vi "build-flow-controller.vi"(10 "Proc Name":string, 11 "Device":T1={"Schedular"={"sched-mode"=enum."Hourly", "sched-pairs"=[]}, "Sensor"={"Input"="ain", "Comparison"=">=", "Setpoint"=0.0}, "Outputs"=[], "Interval"=0, "Timeout"=0, "Mode"=enum."On"} caption="Device Setup" {"Schedular"."sched-pairs"."start" format="%<%H:%M %d/%m>T"; "Schedular"."sched-pairs"."stop" format="%<%H:%M %d/%m>T"; "Timeout" min=1}) -> (3 "Flow":T7[](array[typedef]))   [LabVIEW 2024]
uses:
  controls/UiStepBuilder.ctl
  controls/type.step-builder.ctl
  controls/controller.ctl
  controls/sched-cluster.ctl
  controls/UiScheduleTimestamp.ctl
  controls/UiDeviceSensorParams.ctl
  controls/UiDeviceSensorEquality.ctl
  controls/device-mode.ctl
  controls/typeFlowBuilderDeviceGenerics.ctl
  controls/sched-encoded-cluster.ctl
panel:
  out "error out":errorcluster
  # "Pulse [sec]"
  # "Period [sec]"
  # "Sensor"
  # "Scheduler"
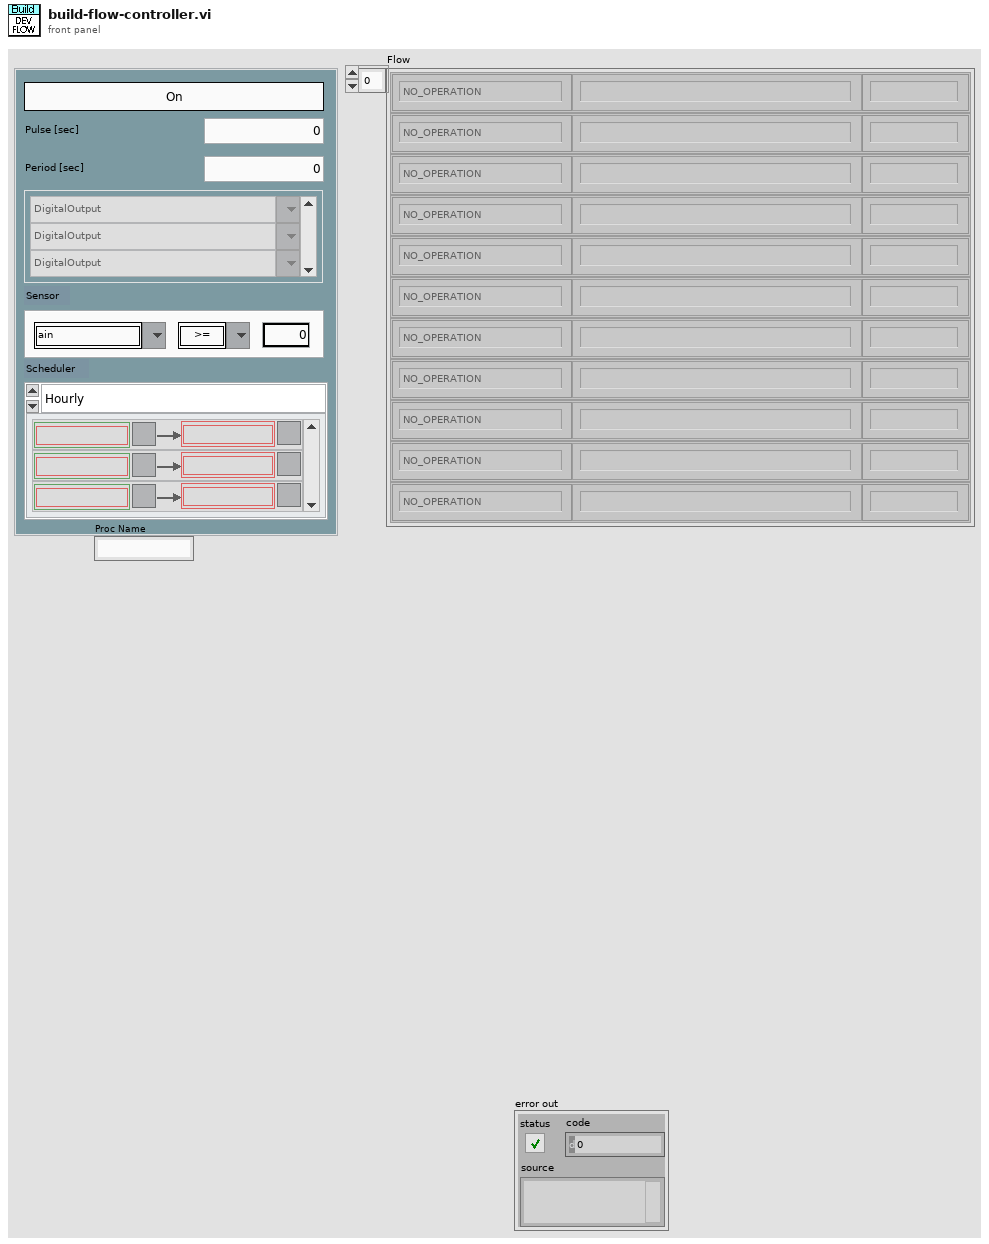
[diagram p1: front panel]
types:
  T1 = typedef "controller.ctl" = cluster{"Schedular":T2, "Sensor":T4, "Outputs":string[], "Interval":u32, "Timeout":u16, "Mode":T6}
  T2 = typedef "sched-cluster.ctl" = cluster{"sched-mode":enum16{"Hourly", "Daily", "Weekly", "Date"}, "sched-pairs":cluster{"start":T3, "stop":T3}[]}
  T3 = typedef "UiScheduleTimestamp.ctl" = timestamp
  T4 = typedef "UiDeviceSensorParams.ctl" = cluster{"Input":string, "Comparison":T5, "Setpoint":dbl}
  T5 = typedef "UiDeviceSensorEquality.ctl" = string
  T6 = typedef "device-mode.ctl" = enum16{"On", "Off", "Sense", "Sched", "Sched AND Sense", "Sched OR Sense"}
  T7 = typedef "UiStepBuilder.ctl" = cluster{"Step Function":T8, "ParamString":string, "Step Label":string}
  T8 = typedef "type.step-builder.ctl" = enum16{"NO_OPERATION", "DELAY-JUMP", "DELAY", "JUMP", "COMPLETE", "SCHEDULER", "IRR-CHECK", "UNIT-CHECK", "UNIT-SAMPLE", "UNIT-DOSE", "LOG-REPORT", "LOG-MESSAGE", "IO-READ", "IO-READ-MANY", "IO-WRITE", "IO-COMPARE-OUT", "IO-COMPARE-IN", "PROC-START", "PROC-STOP", "PROC-LOAD", "PROC-IS-COMPLETED", "RECORD-MOVE", "GET-RH", "GET-UV", "GET-WD", "GET-WS", "OCS-CHECK", "OCS-RECORD"}
  T9 = typedef "typeFlowBuilderDeviceGenerics.ctl" = cluster{"DoutTimeout":u16, "LoopInterval":u32}
  T10 = typedef "sched-encoded-cluster.ctl" = cluster{"StepPtr":string, "SchedPrms":T2}
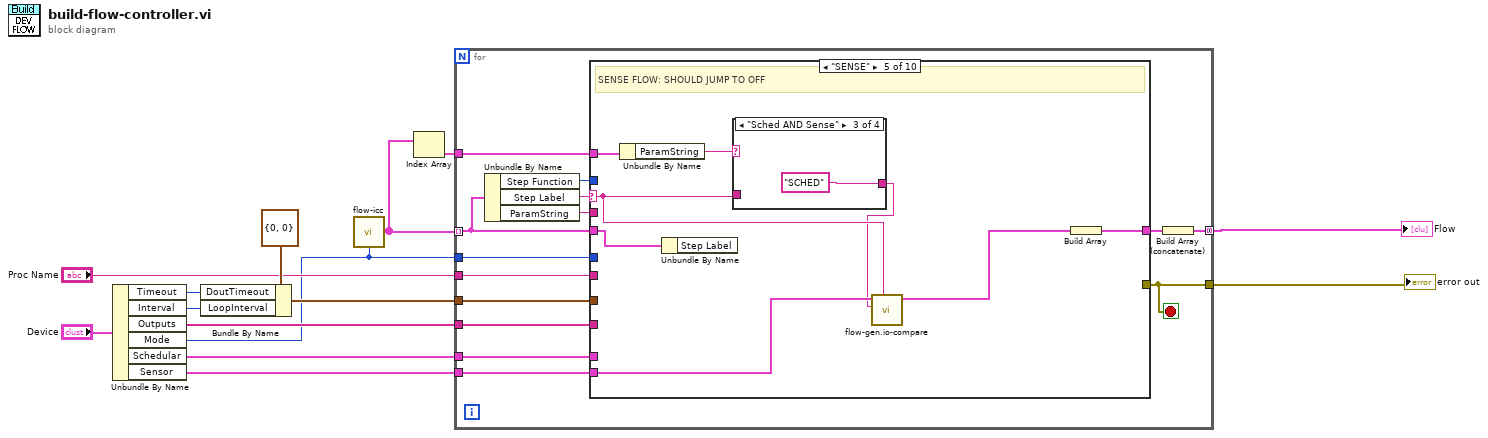
[diagram p0: block diagram]
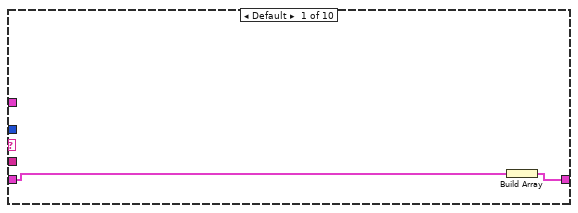
[diagram p2: hidden frame]
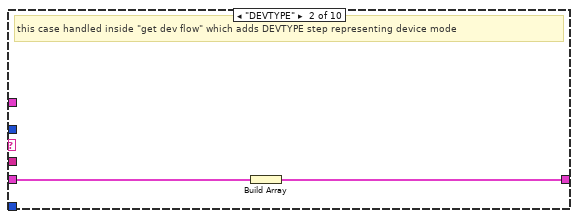
[diagram p3: hidden frame]
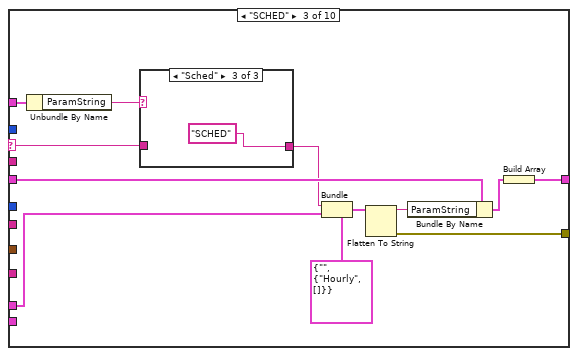
[diagram p4: hidden frame]
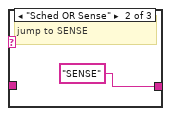
[diagram p6: hidden frame]
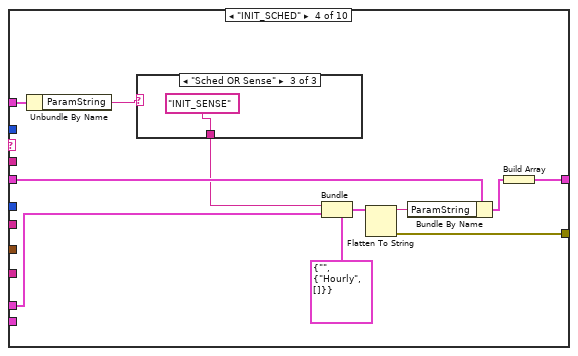
[diagram p7: hidden frame]
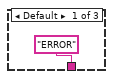
[diagram p8: hidden frame]
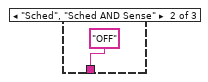
[diagram p9: hidden frame]
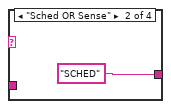
[diagram p11: hidden frame]
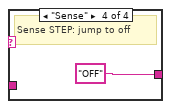
[diagram p12: hidden frame]
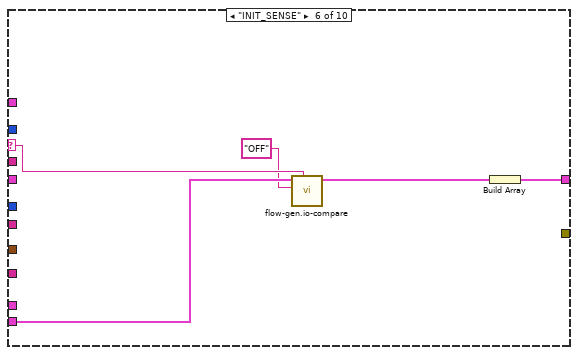
[diagram p13: hidden frame]
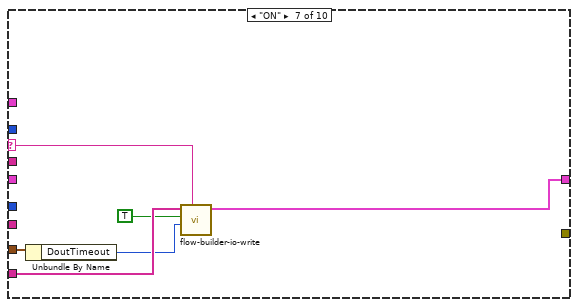
[diagram p14: hidden frame]
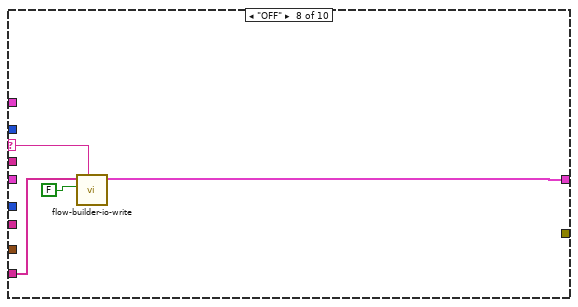
[diagram p15: hidden frame]
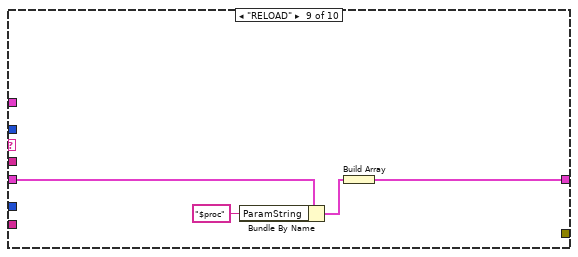
[diagram p16: hidden frame]
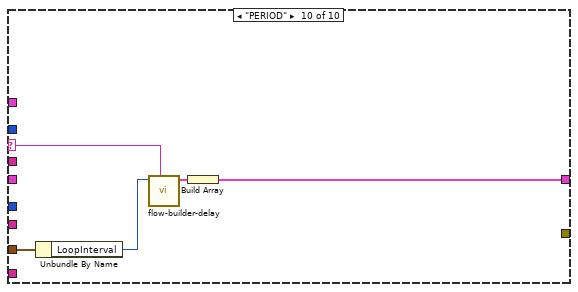
[diagram p17: hidden frame]
diagram:
  n1 = Unbundle By Name("Device") -> ("Timeout"=w11:u16, "Interval"=w12:u32, "Outputs"=w13:string[], "Mode"=w5:T6, "Schedular"=w2:T2, "Sensor"=w1:T4)
  n2 = Bundle By Name(cluster=T9 {"DoutTimeout"=0, "LoopInterval"=0} ("Device General Params"), "DoutTimeout"=w11, "LoopInterval"=w12) -> (w8:T9)
  n3 = call "flow-icc.vi"("Mode"=w5) -> ("ICC Flow Templates"=w4:T7[])  [unwired: 10 in]
  n4 = Index Array(array=w4) -> (element=w3:T7)  [unwired: 1 in]
  n5 = for {
    tunnel: w4 -> [w27] mode=indexing
    tunnel: [w24] -> w14 mode=concatenating
    tunnel: w8 -> [w25]
    tunnel: w13 -> [w23]
    tunnel: "Proc Name" -> [w20]
    tunnel: w5 -> [w19]
    tunnel: [w18] -> w7
    tunnel: w3 -> [w17]
    tunnel: w2 -> [w16]
    tunnel: w1 -> [w15]
    stop <- w18 stop-if-true
    n6 = Unbundle By Name(w27) -> ("Step Function"=w21:T8, "Step Label"=w28:string, "ParamString"=w22:string)
    n7 = case shown="\"SENSE\"" w28 {
      selector: w28 -> [_ _ w35 _ w64 w75 w81 w86 _ w95]
      tunnel: w27 -> [w30 w32 w43 w57 w62 _ _ _ w91 _]
      tunnel: [w29 w31 w44 w58 w68 w77 w84 w88 w92 w93] -> w26
      tunnel: w25 -> [_ _ _ _ _ _ w83 _ _ w97]
      tunnel: w23 -> [_ _ _ _ _ _ w82 w87 _ _]
      tunnel: w22 -> [_ _ _ _ _ _ _ _ _ _]
      tunnel: w21 -> [_ _ _ _ _ _ _ _ _ _]
      tunnel: w20 -> [_ _ _ _ _ _ _ _ _ _]
      tunnel: w19 -> [_ _ _ _ _ _ _ _ _ _]
      tunnel: [_ _ w40 w54 _ _ _ _ _ _] -> w18
      tunnel: w17 -> [_ _ w37 w51 w65 _ _ _ _ _]
      tunnel: w16 -> [_ _ w33 w50 _ _ _ _ _ _]
      tunnel: w15 -> [_ _ _ _ w67 w76 _ _ _ _]
      frame Default {
        n8 = Build Array(w30) -> (w29:T7[])
      }
      frame "DEVTYPE" {
        # "this case handled inside \"get dev flow\" which adds DEVTYPE step representing device mode"
        n9 = Build Array(w32) -> (w31:T7[])
      }
      frame "SCHED" {
        n10 = Unbundle By Name(w37) -> ("ParamString"=w36:string)
        n11 = case shown="\"Sched\"" w36 {
          tunnel: w35 -> [w45 _ _]
          tunnel: [w45 "SENSE" "SCHED"] -> w34
          frame Default {
            # "self loop"
          }
          frame "Sched OR Sense" {
            # "jump to SENSE"
          }
          frame "Sched" {
          }
        }
        n12 = Bundle(cluster=T10 {"StepPtr"="", "SchedPrms"={"sched-mode"=enum."Hourly", "sched-pairs"=[]}}, "StepPtr"=w34, "SchedPrms"=w33) -> (w41:T10)
        n13 = Flatten To String(anything=w41) -> (data string=w38:string, error out=w40:errorcluster)  [unwired: 3 in, 1 out]
        n14 = Bundle By Name(cluster=w43, "ParamString"=w38) -> (w42:T7)
        n15 = Build Array(w42) -> (w44:T7[])
      }
      frame "INIT_SCHED" {
        n16 = Unbundle By Name(w51) -> ("ParamString"=w48:string)
        n17 = case shown="\"Sched OR Sense\"" w48 {
          tunnel: ["ERROR" "OFF" "INIT_SENSE"] -> w49
          frame Default {
          }
          frame "Sched", "Sched AND Sense" {
          }
          frame "Sched OR Sense" {
          }
        }
        n18 = Bundle(cluster=T10 {"StepPtr"="", "SchedPrms"={"sched-mode"=enum."Hourly", "sched-pairs"=[]}}, "StepPtr"=w49, "SchedPrms"=w50) -> (w55:T10)
        n19 = Flatten To String(anything=w55) -> (data string=w52:string, error out=w54:errorcluster)  [unwired: 3 in, 1 out]
        n20 = Bundle By Name(cluster=w57, "ParamString"=w52) -> (w56:T7)
        n21 = Build Array(w56) -> (w58:T7[])
      }
      frame "SENSE" {
        # "SENSE FLOW: SHOULD JUMP TO OFF"
        n22 = Unbundle By Name(w65) -> ("ParamString"=w66:string)
        n23 = Unbundle By Name(w62) -> ()  [unwired: 1 out]
        n24 = case shown="\"Sched AND Sense\"" w66 {
          tunnel: w64 -> [w70 _ _ _]
          tunnel: [w70 "SCHED" "SCHED" "OFF"] -> w63
          frame Default {
            # "self loop"
          }
          frame "Sched OR Sense" {
          }
          frame "Sched AND Sense" {
          }
          frame "Sense" {
            # "Sense STEP: jump to off"
          }
        }
        n25 = call "flow-gen.io-compare.vi"("Step Label"=w64, "stepPointer (False Cond.)"=w63, "Device Sensor Params"=w67) -> ("Step out"=w69:T7)  [unwired: 8 in]
        n26 = Build Array(w69) -> (w68:T7[])
      }
      frame "INIT_SENSE" {
        n27 = call "flow-gen.io-compare.vi"("Step Label"=w75, "stepPointer (False Cond.)"="OFF", "Device Sensor Params"=w76) -> ("Step out"=w78:T7)  [unwired: 8 in]
        n28 = Build Array(w78) -> (w77:T7[])
      }
      frame "ON" {
        n29 = Unbundle By Name(w83) -> ("DoutTimeout"=w79:u16)
        n30 = call "flow-builder-io-write.vi"("Step Name"=w81, "Digital Timeout"=w79, "Value in"=TRUE ("UiDeviceConstant"), "Dout+AUX"=w82) -> ("Flow out"=w84:T7[])  [unwired: 7 in]
      }
      frame "OFF" {
        n31 = call "flow-builder-io-write.vi"("Step Name"=w86, "Value in"=FALSE ("UiDeviceConstant"), "Dout+AUX"=w87) -> ("Flow out"=w88:T7[])  [unwired: 8 in]
      }
      frame "RELOAD" {
        n32 = Bundle By Name(cluster=w91, "ParamString"="$proc") -> (w90:T7)
        n33 = Build Array(w90) -> (w92:T7[])
      }
      frame "PERIOD" {
        n34 = Unbundle By Name(w97) -> ("LoopInterval"=w96:u32)
        n35 = call "flow-builder-delay.vi"("Step Label"=w95, "Delay [s]"=w96) -> ("Step Element"=w94:T7)  [unwired: 9 in]
        n36 = Build Array(w94) -> (w93:T7[])
      }
    }
    n37 = Build Array (concatenate)(w26) -> (w24:T7[])
  }
  "Flow" <- w14
  "error out" <- w7
